vi "工具-生成状态订阅图.vi"() -> ()   [LabVIEW 2020]
uses:
  <vilib>/sklein/WebView2/Webview2 Control/WebView2 Control.xctl
  <vilib>/httpClient/LabVIEWHTTPClient.lvlib
  <userlib>/_NEVSTOP/Communicable State Machine(CSM)/Communicable State Machine.lvlib
  <vilib>/httpClient/POSTBuffer.vi
  <vilib>/Utility/sysdir.llb/System Directory Type.ctl
  <vilib>/sklein/WebView2/Webview2 Control/Paths.ctl
panel:
  out "Timed Out":bool
  out "URL":string="http://ni.com"
  in  "Go":bool
  out "Status":string
  out "resulting string 3":string
  out "resulting string 2":string
  out "Chart":string(xcontrol)
  # "https://mermaid.live/"
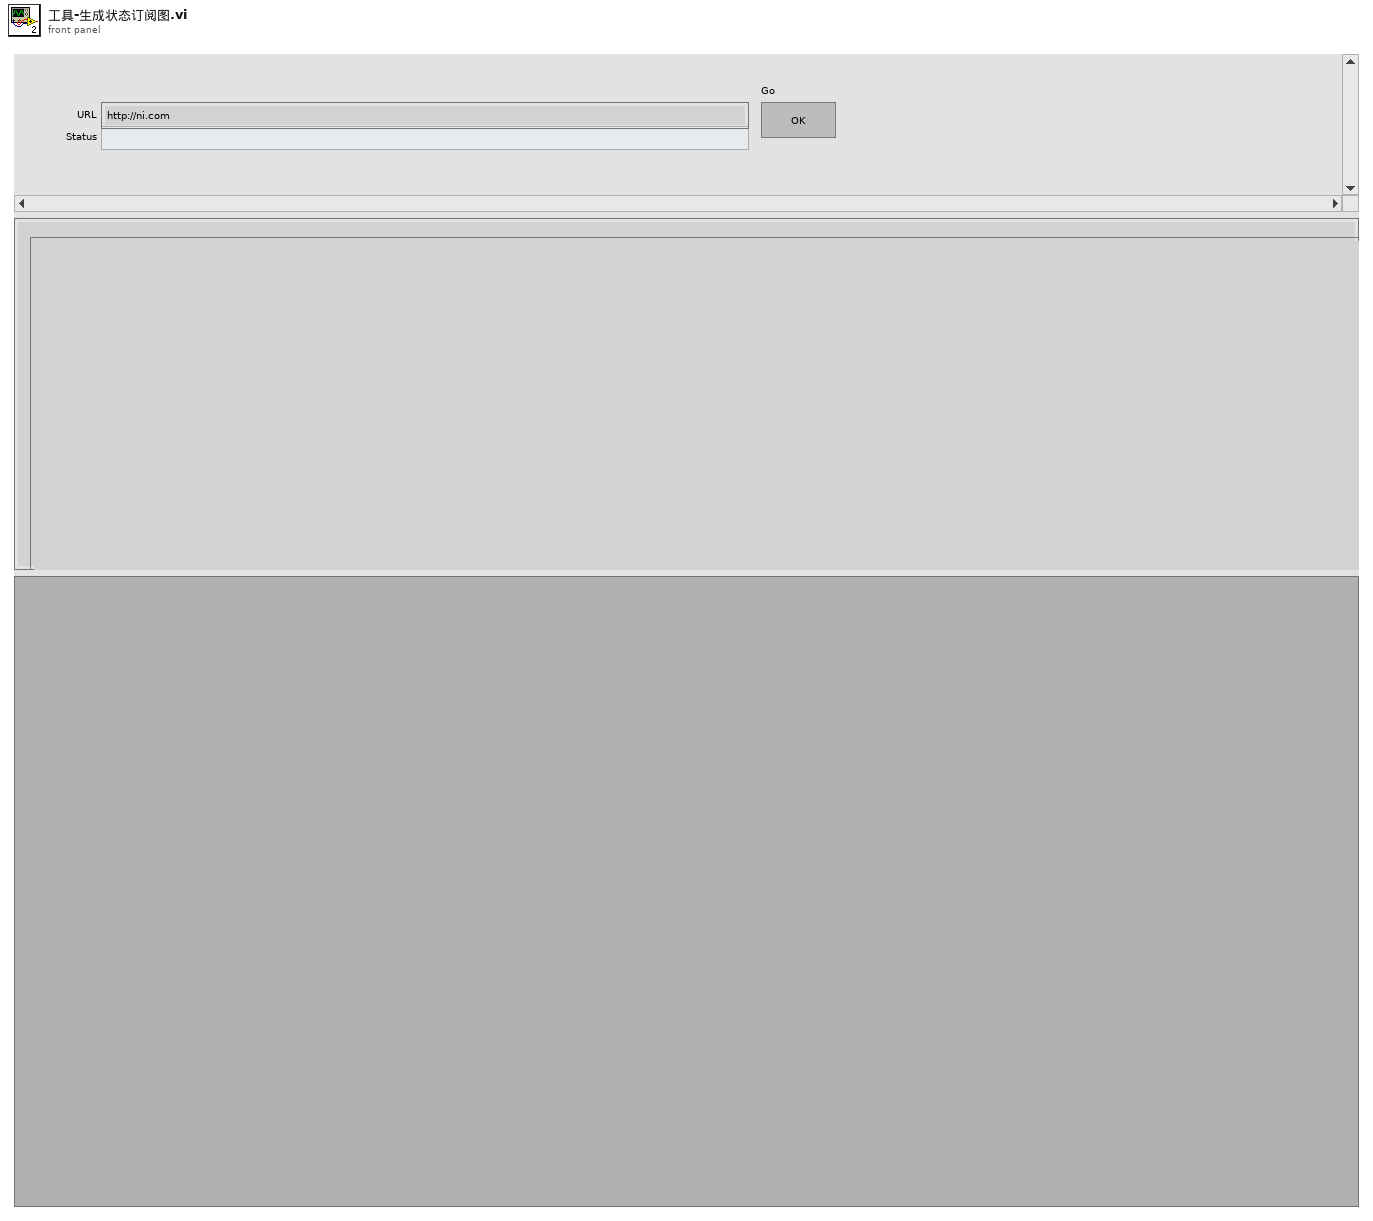
[diagram p1: front panel]
types:
  T1 = typedef "WebView2 Control.xctl/Paths.ctl" = cluster{"Webview2 Native":path, "Edge Application":path, "User Data":path}
  T2 = typedef "System Directory Type.ctl" = i32
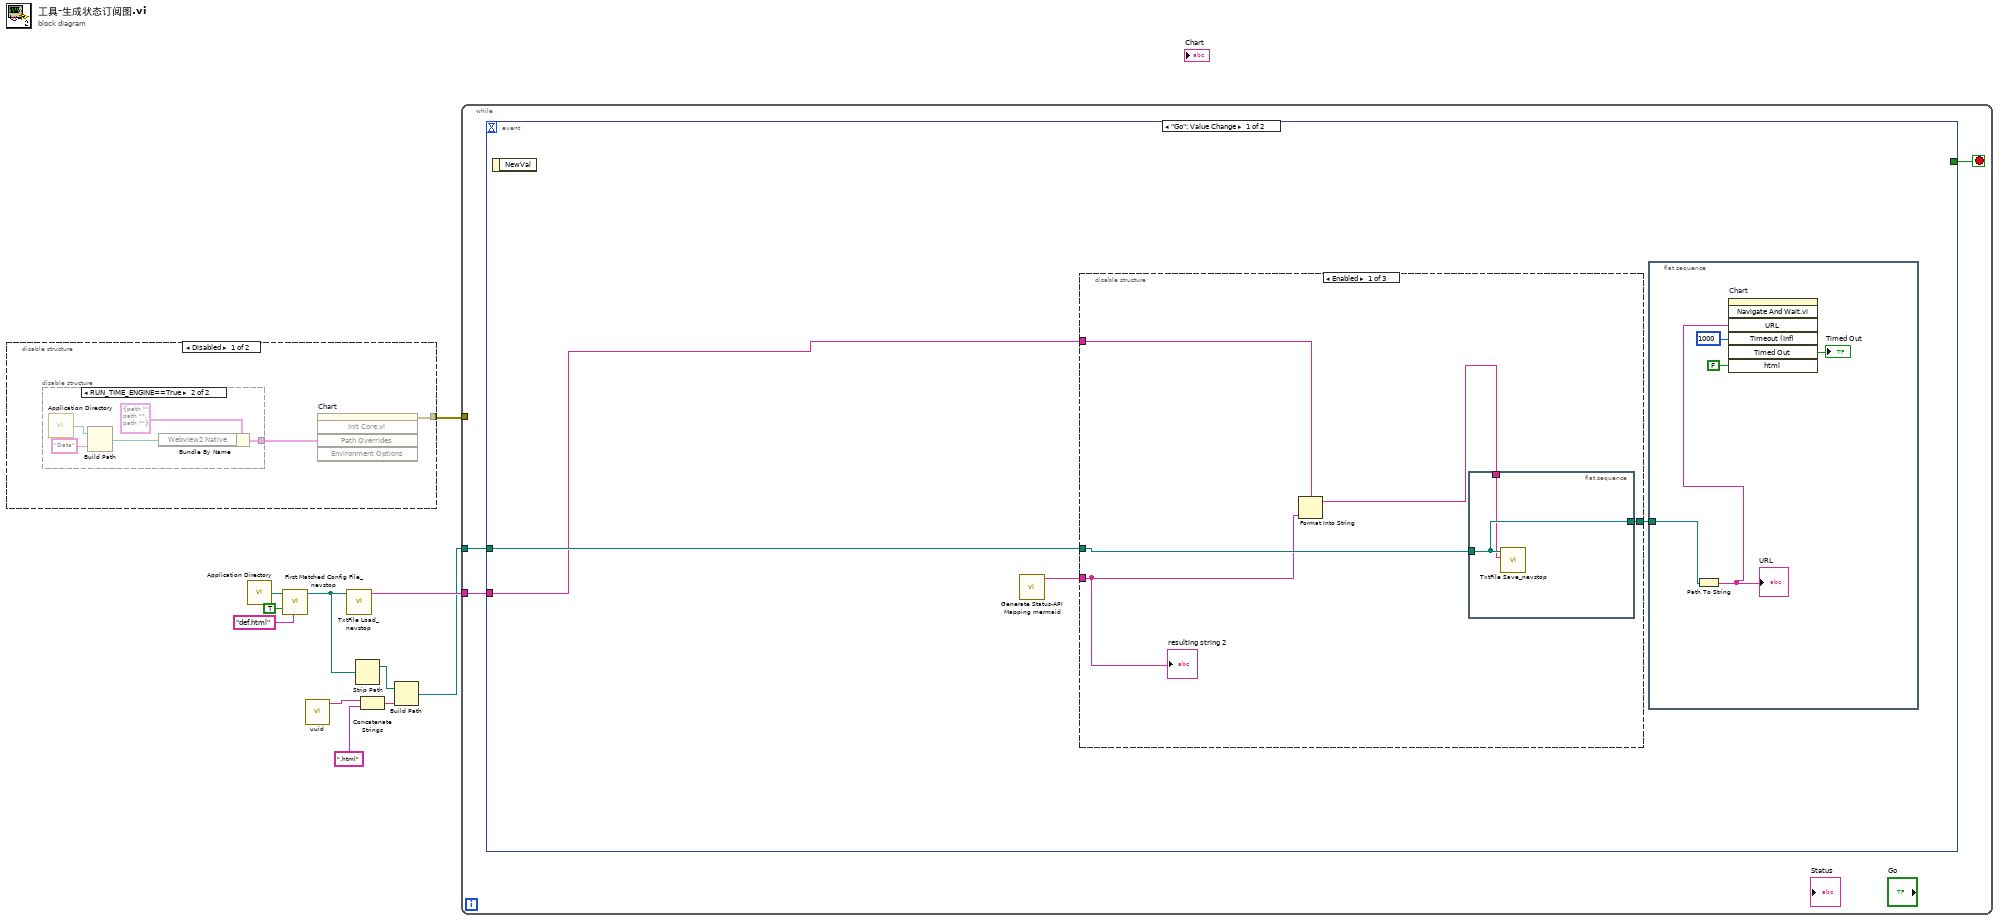
[diagram p0: block diagram]
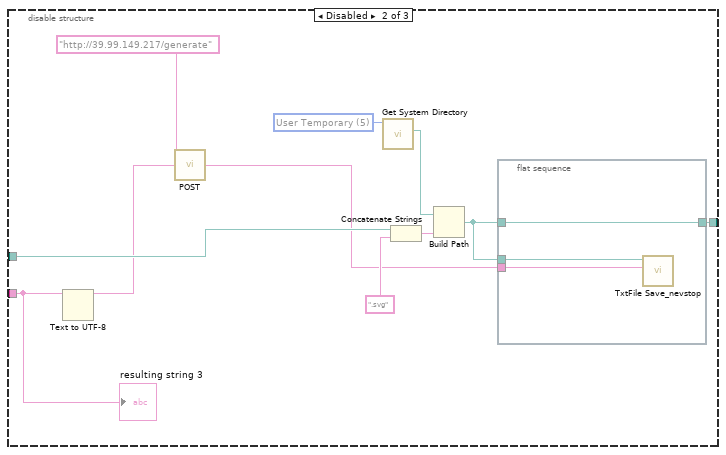
[diagram p4: hidden frame]
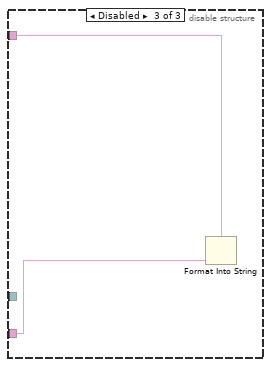
[diagram p5: hidden frame]
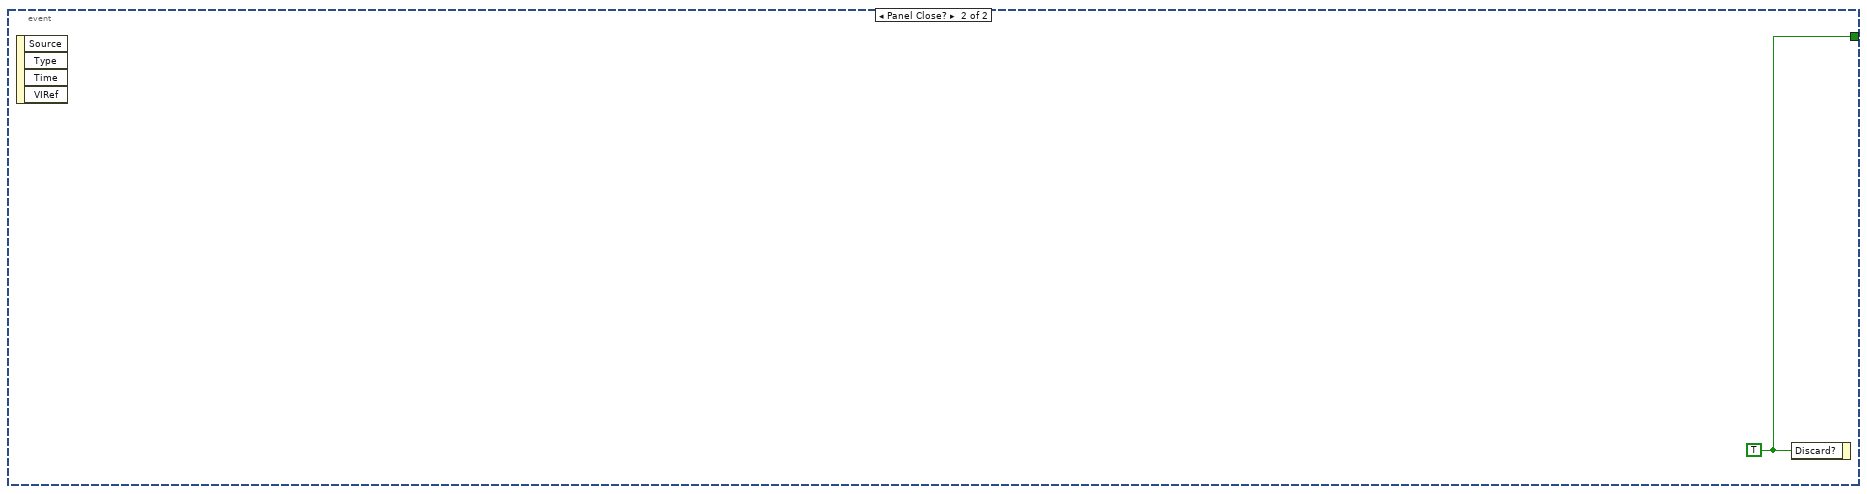
[diagram p6: hidden frame]
diagram:
  n1 = disable-structure shown="Disabled" {
    disable-tunnel: [w12 _] -> w11
    frame Disabled {
      n2 = disable-structure shown="RUN_TIME_ENGINE==True" {
        disable-tunnel: [_ w17] -> w13
        frame condition #0 (active) {
        }
        frame condition #1 {
          n3 = call <vilib>:"Application Directory.vi"() -> ("Application Directory"=w15:path)
          n4 = Build Path(base path=w15, name or relative path="Data") -> (appended path=w16:path)
          n5 = Bundle By Name(cluster=T1 {"Webview2 Native"=path "", "Edge Application"=path "", "User Data"=path ""} ("Path Overrides"), "Webview2 Native"=w16) -> (w17:T1)
        }
      }
      n6 = invoke on="Chart" class="WebView2 Control (strict)" method="Init Core.vi"("Path Overrides"=w13) -> (error out=w12:errorcluster)  [unwired: 4 in, 4 out]
    }
    frame Enabled {
    }
  }
  n7 = call <vilib>:"Application Directory.vi"() -> ("Application Directory"=w10:path)
  n8 = call <userlib>:"First Matched Config File_nevstop.vi"("pattern(ini by default)"="def.html", "Recrusively(F)"=TRUE, "Searching Directory"=w10) -> ("Matched Config File"=w6:path)  [unwired: 8 in]
  n9 = call <userlib>:"uuid.vi"() -> ("UUID"=w2:string)  [unwired: 11 in]
  n10 = call <userlib>:"TxtFile Load_nevstop.vi"("Path"=w6) -> ("text"=w7:string)  [unwired: 9 in, 1 out]
  n11 = Strip Path(path=w6) -> (stripped path=w3:path)  [unwired: 1 out]
  n12 = Concatenate Strings(w2, ".html" ("string")) -> (w4:string)
  n13 = Build Path(base path=w3, name or relative path=w4) -> (appended path=w1:path)
  n14 = while {
    tunnel: w1 -> [w20]
    tunnel: w11 -> [_]
    tunnel: w7 -> [w19]
    stop <- w21 stop-if-true
    n15 = event shown="[0] \"Go\": Value Change" {
      selector: _ -> [_ _]
      dyn-events: _ -> [_ _]
      timeout: _ -> [_ _]
      tunnel: [_ w54] -> w21
      tunnel: w20 -> [w23 _]
      tunnel: w19 -> [w22 _]
      event "Go": Value Change {
        n16 = event-data() -> ()  [unwired: 1 in, 1 out]
        n17 = call "Generate Status-API Mapping mermaid.vi"() -> ("String"=w25:string)  [unwired: 10 in, 1 out]
        n18 = disable-structure "Diagram Disable Structure" shown="Enabled" {
          disable-tunnel: w25 -> [w26 w42 w47]
          disable-tunnel: [w30 w39 _] -> w24
          disable-tunnel: w23 -> [w29 w37 _]
          disable-tunnel: w22 -> [w28 _ w48]
          frame Enabled {
            n19 = Format Into String(format string=w28, w26) -> (resulting string=w27:string)  [unwired: 2 in, 1 out]
            n20 = flat-sequence {
              tunnel: [w32] -> _
              tunnel: [w32] -> w30
              tunnel: w29 -> [w32]
              tunnel: w27 -> [w31]
              frame #0 {
                n21 = call <userlib>:"TxtFile Save_nevstop.vi"("text"=w31, "Path"=w32) -> ()  [unwired: 9 in, 1 out]
              }
            }
            "resulting string 2" <- w26
          }
          frame Disabled {
            w36 = T2 5 items=["User Home"=0, "User Desktop"=1, "User Documents"=2, "User Application Data"=3, "User Preferences"=4, "User Temporary"=5, "Public Documents"=6, "Public Application Data"=7, "Public Preferences"=8, "Public Cache"=13, "System Core Libraries"=9, "System Installed Libraries"=10, "Application Files"=11, "Boot Volume Root"=12] ("system directory type")
            n22 = Text to UTF-8(11:w42) -> (3:w34:string)  [unwired: 2 in, 1 out]
            n23 = call-poly <vilib>:"POST.vi"("url"="http://39.99.149.217/generate", "buffer"=w34) -> ("body"=w33:string)  [unwired: 10 in, 3 out]
            n24 = call <vilib>:"Get System Directory.vi"("system directory type"=w36) -> ("system directory"=w35:path)  [unwired: 10 in]
            n25 = Concatenate Strings(w37, ".svg" ("string")) -> (w43:string)
            n26 = Build Path(base path=w35, name or relative path=w43) -> (appended path=w38:path)
            n27 = flat-sequence {
              tunnel: w33 -> [w44]
              tunnel: w38 -> [w46]
              tunnel: [w45] -> w39
              tunnel: w38 -> [w45]
              frame #0 {
                n28 = call <userlib>:"TxtFile Save_nevstop.vi"("text"=w44, "Path"=w46) -> ()  [unwired: 9 in, 1 out]
              }
            }
            "resulting string 3" <- w42
          }
          frame Disabled {
            n29 = Format Into String(format string=w48, w47) -> ()  [unwired: 2 in, 2 out]
          }
        }
        n30 = flat-sequence {
          tunnel: w24 -> [w53]
          frame #0 {
            n31 = Path To String(path=w53) -> (string=w49:string)
            "URL" <- w49
            n32 = invoke on="Chart" class="WebView2 Control (strict)" method="Navigate And Wait.vi"("URL"=w49, "Timeout (Inf)"=1000, "html"=FALSE) -> ("Timed Out"=→"Timed Out":bool)  [unwired: 4 in, 6 out]
          }
        }
      }
      event Panel Close? {
        w54 = TRUE ("Discard?")
        n33 = event-data() -> ()  [unwired: 1 in, 4 out]
        n34 = event-data("Discard?"=w54) -> ()  [unwired: 1 in, 1 out]
      }
    }
  }
